vi "Main.vi"(8 "error in (no error)":errorcluster, 11 "Process in":refnum<class "Random Process.lvclass">) -> (0 "error out":errorcluster, 3 "Process out":refnum<class "Random Process.lvclass">)   [LabVIEW 2019, in "TelemetryAsync Engine.lvlib" / "Random Process.lvclass"]
uses:
  Random Process.lvclass
  C:/Users/XEnderMD/Desktop/CD Project Tools/Source/Engine/Parent Classes/Process/Process.lvclass
  Parent Classes/Process/Process.lvclass/Process.ctl
  <vilib>/Platform/TimedLoop/XDataNode/timing_clust.ctl
  <vilib>/Platform/TimedLoop/XDataNode/nitl_modes.ctl
  <vilib>/Platform/TimedLoop/XDataNode/wakeup.ctl
  <vilib>/platform/TimedLoop/XDataNode/XDataNode.xnode
  Parent Classes/Process/Process.lvclass
  <vilib>/NI VeriStand/Custom Device API/Custom Device API.lvlib
  <vilib>/Platform/TimedLoop/XDataNode/XDNodeRunTimeDep.lvlib
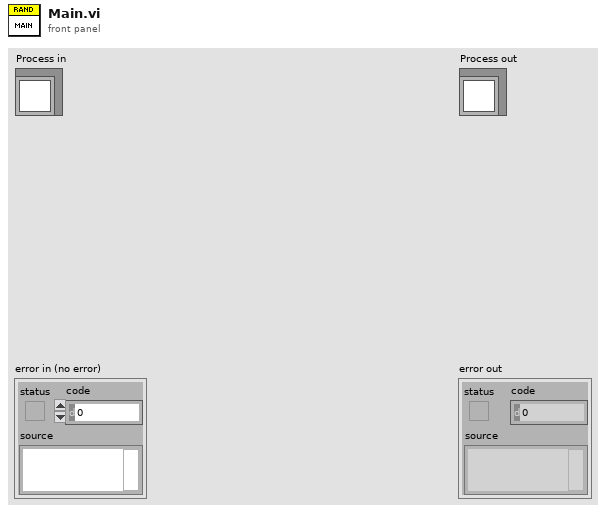
[diagram p1: front panel]
types:
  T1 = typedef "XDNodeRunTimeDep.lvlib/timing_clust.ctl" = cluster{"Expected End [f-1]":u64, "Actual End [f-1]":u64, "Finished Late? [f-1]":bool, "Expected End [i-1]":u64, "Actual End [i-1]":u64, "Finished Late? [i-1]":bool, "Expected Start [i]":u64, "Actual Start [i]":u64, "Expected Start [f]":u64, "Actual Start [f]":u64, "Source Name":string, "Structure Name":string, "Period":i64, "Deadline":i64, "Offset":i64, "Start":i64, "Priority":i32, "Timeout":i32, "Mode":T2, "Wakeup Reason":T3, "Error":errorcluster, "Source Type":string, "Secondary Source Type":string, "Global End Time":u64, "Global Start Time":u64, "Frame Duration":u64, "Iteration Duration":u64, "Assigned CPU":i32, "I/O Scan Engine Mode":u32}
  T2 = typedef "XDNodeRunTimeDep.lvlib/nitl_modes.ctl" = enum32{"No Change", "Process missed periods, maintain original phase", "Discard missed periods, maintain original phase", "Process missed periods, ignore original phase", "Discard missed periods, ignore original phase"}
  T3 = typedef "XDNodeRunTimeDep.lvlib/wakeup.ctl" = enum32{"Normal", "Aborted", "Asynchronous wakeup", "Timing source error", "Timed loop error", "Timeout"}
  T4 = typedef "TelemetryAsync Engine.lvlib/Process.lvclass/Async Paramters.ctl" = cluster{"Device Reference":T5, "Device Clock":string, "Device Inputs FIFO":refnum<k33>, "Device Outputs FIFO":refnum<k33>, "CD Engine Event Ref":T6}
  T5 = typedef "Custom Device API.lvlib/Custom Device Item Ref.ctl" = u64
  T6 = typedef "Custom Device API.lvlib/Custom Device Engine Event Ref.ctl" = refnum<event-registration>
  T7 = typedef "Custom Device API.lvlib/Custom Device Timed Loop Priority.ctl" = enum32{"Low", "Medium", "High"}
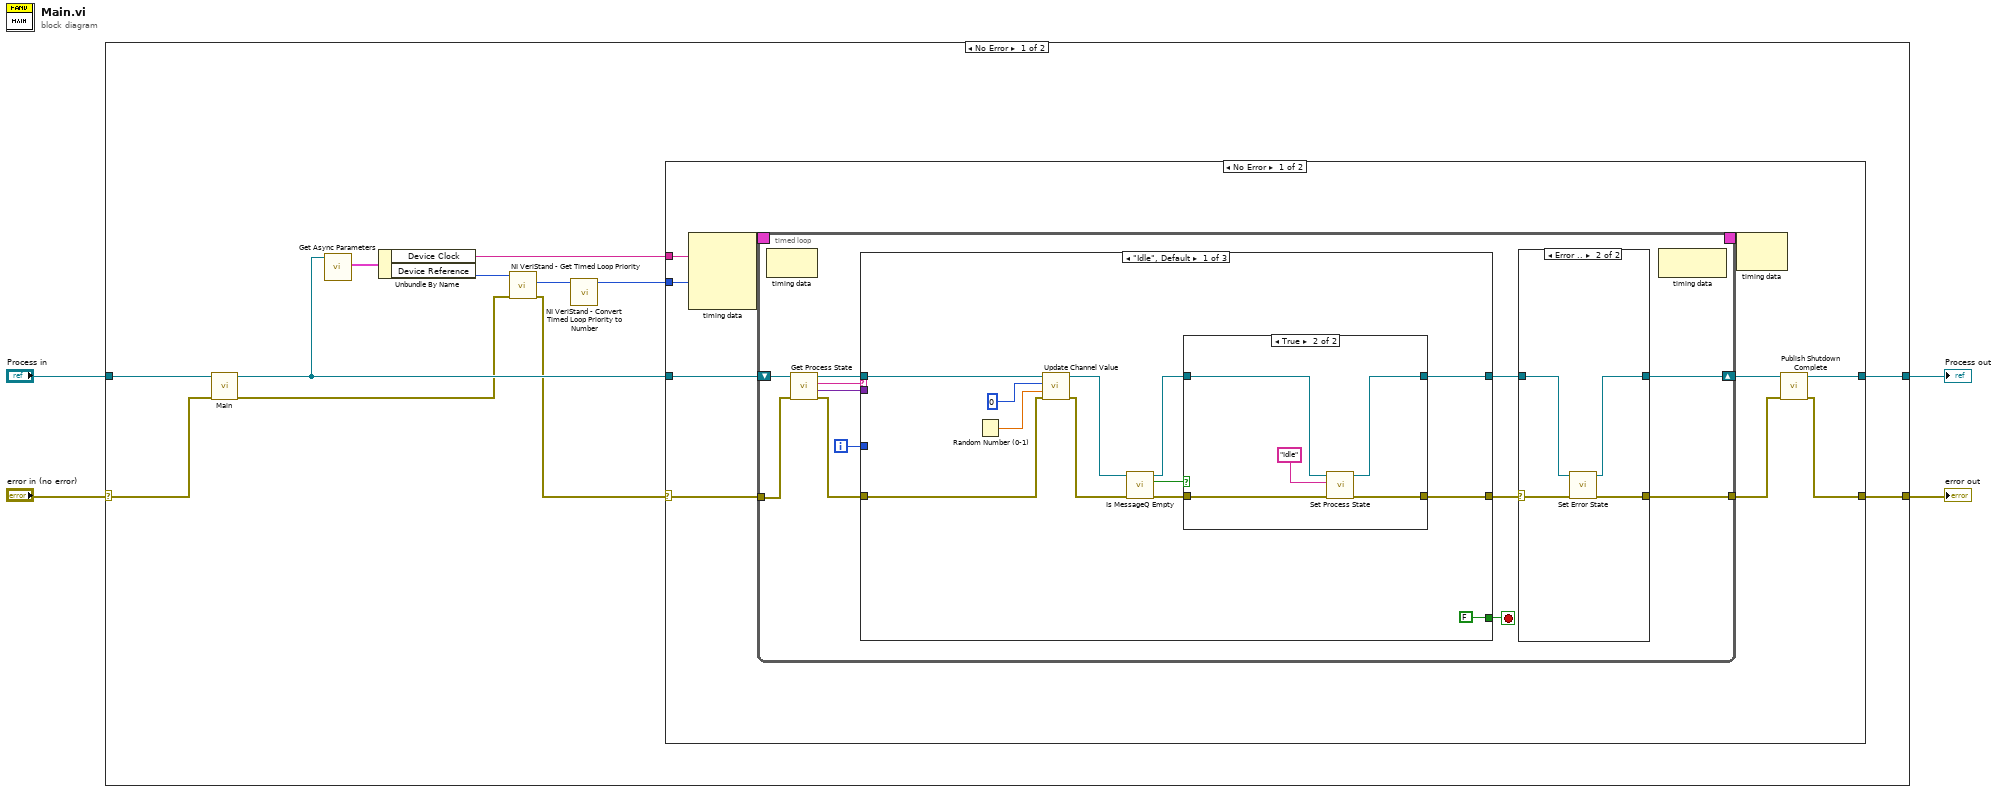
[diagram p0: block diagram]
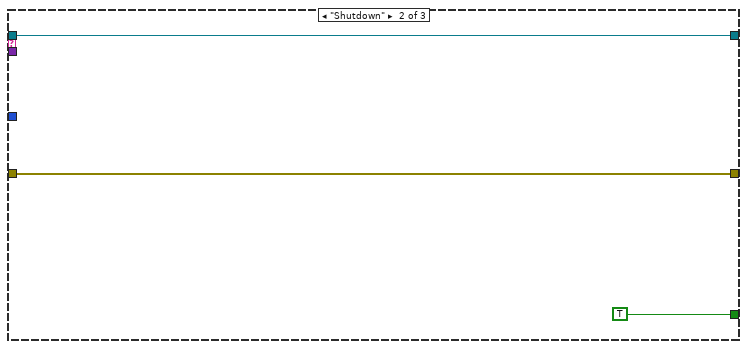
[diagram p4: hidden frame]
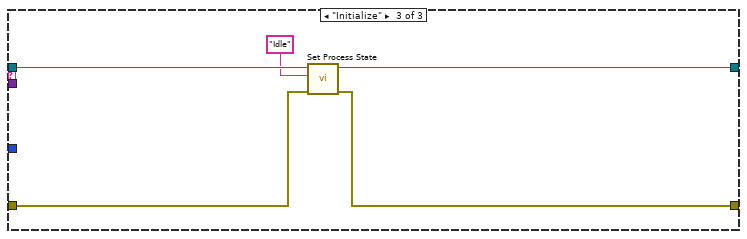
[diagram p5: hidden frame]
diagram:
  n1 = case shown="No Error" "error in (no error)" {
    selector: "error in (no error)" -> [w15 w82]
    tunnel: [w13 w82] -> w1
    tunnel: [w14 w81] -> w2
    tunnel: "Process in" -> [w16 w81]
    frame No Error {
      n2 = call-parent "Main.vi"("error in (no error)"=w15, "Process in"=w16) -> ("error out"=w7:errorcluster, "Process out"=w10:refnum<class "Random Process.lvclass">)  [unwired: 8 in]
      n3 = call "Get Async Parameters.vi"("Process in"=w10) -> ("Async Parameters"=w12:T4)  [unwired: 9 in, 1 out]
      n4 = Unbundle By Name(w12) -> ("Device Clock"=w9:string, "Device Reference"=w11:T5)
      n5 = call <vilib>:"NI VeriStand - Get Timed Loop Priority.vi"("error in (no error)"=w7, "Device Ref in"=w11) -> ("error out"=w5:errorcluster, "Priority"=w8:T7)  [unwired: 7 in, 1 out]
      n6 = call <vilib>:"NI VeriStand - Convert Timed Loop Priority to Number.vi"("Priority"=w8) -> ("Numeric Priority"=w6:i32)  [unwired: 10 in]
      n7 = case shown="No Error" w5 {
        selector: w5 -> [w18 w79]
        tunnel: [w23 w80] -> w14
        tunnel: [w21 w79] -> w13
        tunnel: w9 -> [w20 _]
        tunnel: w10 -> [w19 w80]
        tunnel: w6 -> [w17 _]
        frame No Error {
          n8 = node-c288(w20, w17) -> (w26:T1)  [unwired: 2 in]
          n9 = timed-loop {
            shift-right: [w31] -> w24
            shift-left: w19 -> [w37]
            tunnel: w18 -> [w38]
            tunnel: [w30] -> w22
            timing: w26 -> [_]
            timing-out: [_] -> w25
            i -> [w27]
            stop <- w29 stop-if-true
            n10 = node-c288() -> ()  [unwired: 1 in, 1 out]
            n11 = call "Get Process State.vi"("error in (no error)"=w38, "Process in"=w37) -> ("error out"=w34:errorcluster, "Payload"=w35:variant, "Command"=w28:string, "Process out"=w36:refnum<class "Random Process.lvclass">)  [unwired: 6 in]
            n12 = case shown="\"Idle\", Default" w28 {
              tunnel: w36 -> [w57 w68 w73]
              tunnel: w35 -> [_ _ _]
              tunnel: w34 -> [w56 w67 w72]
              tunnel: [w49 w68 w71] -> w33
              tunnel: [w48 w67 w70] -> w32
              tunnel: [FALSE TRUE _] -> w29
              tunnel: w27 -> [_ _ _]
              frame "Idle", Default {
                n13 = Random Number (0-1)() -> (number: 0 to 1=w47:dbl)
                n14 = call "Update Channel Value.vi"("error in (no error)"=w56, "New Value"=w47, "Channel Index"=0, "Output Process in"=w57) -> ("error out"=w54:errorcluster, "Output Process out"=w53:refnum<class "Random Process.lvclass">)  [unwired: 4 in, 2 out]
                n15 = call "Is MessageQ Empty.vi"("error in (no error)"=w54, "Process in"=w53) -> ("error out"=w51:errorcluster, "is Empty ?"=w52:bool, "Process out"=w50:refnum<class "Random Process.lvclass">)  [unwired: 7 in]
                n16 = case shown="True" w52 {
                  tunnel: w51 -> [w59 w61]
                  tunnel: w50 -> [w60 w64]
                  tunnel: [w60 w63] -> w49
                  tunnel: [w59 w62] -> w48
                  frame False {
                  }
                  frame True {
                    n17 = call "Set Process State.vi"("error in (no error)"=w61, "Command"="Idle", "Process in"=w64) -> ("error out"=w62:errorcluster, "Process out"=w63:refnum<class "Random Process.lvclass">)  [unwired: 7 in]
                  }
                }
              }
              frame "Shutdown" {
              }
              frame "Initialize" {
                n18 = call "Set Process State.vi"("error in (no error)"=w72, "Command"="Idle", "Process in"=w73) -> ("error out"=w70:errorcluster, "Process out"=w71:refnum<class "Random Process.lvclass">)  [unwired: 7 in]
              }
            }
            n19 = case shown="Error .." w32 {
              selector: w32 -> [w41 w46]
              tunnel: w33 -> [w42 w45]
              tunnel: [w42 w44] -> w31
              tunnel: [w41 w43] -> w30
              frame No Error {
              }
              frame Error {
                n20 = call "Set Error State.vi"("error in (no error)"=w46, "Process in"=w45) -> ("error out"=w43:errorcluster, "Process out"=w44:refnum<class "Random Process.lvclass">)  [unwired: 8 in]
              }
            }
            n21 = node-c288() -> ()  [unwired: 1 in, 1 out]
          }
          n22 = node-c288(w25) -> ()  [unwired: 1 out]
          n23 = call "Publish Shutdown Complete.vi"("error in (no error)"=w22, "Process in"=w24) -> ("error out"=w21:errorcluster, "Process out"=w23:refnum<class "Random Process.lvclass">)  [unwired: 8 in]
        }
        frame Error {
        }
      }
    }
    frame Error {
    }
  }
  "error out" <- w1
  "Process out" <- w2
